vi "Define Customized Character.vi"   [LabVIEW 2015, in "HD44780 Host.lvlib"]
doc: "Customizes characters on character LCD devices."
uses:
  HD44780 Host.lvlib
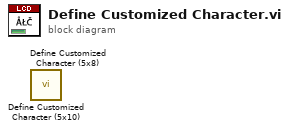
[diagram p0: block diagram]
diagram:
  n1 = call "Define Customized Character (5x10).vi"() -> ()  [unwired: 9 in, 3 out]
  n2 = call "Define Customized Character (5x8).vi"() -> ()  [unwired: 9 in, 3 out]
